vi "Save into new sequence.vi"(5 "To":u32, 7 "From":u32, 9 "Header2 file data":T1, 10 "Header file data":T2 {"Pixel depth" items=["8 bits", "16 bits", "Float", "Complex", "RGB", "HSL"]; "time of 1st frame, \nsec since 1/1/04" format="%.2f"}, 11 "Acquisition refnum array":refnum<file>[](array[refnum])) -> ()   [LabVIEW 2015]
uses:
  GLIMPSE Globals.vi
  Seq file v 1/Offset.ctl
  Seq file v 1/file number.ctl
  Seq file v 1/Offset table.ctl
  Header file data.ctl
  Header2 file data.ctl
panel:
  out "Output frame number 2":i32(slide) scale=0.0..68.0
  out "Input Sequences Progress (%) 2":dbl[](array[slide]) scale=0.0..100.0
  in  "error in":errorcluster
  out "Input Sequences Progress (%)":dbl[](array[slide]) scale=0.0..100.0
  out "Output frame number":i32(slide) scale=0.0..68.0
  out "Save into new directory:":path=path "d:/1.glimpse"
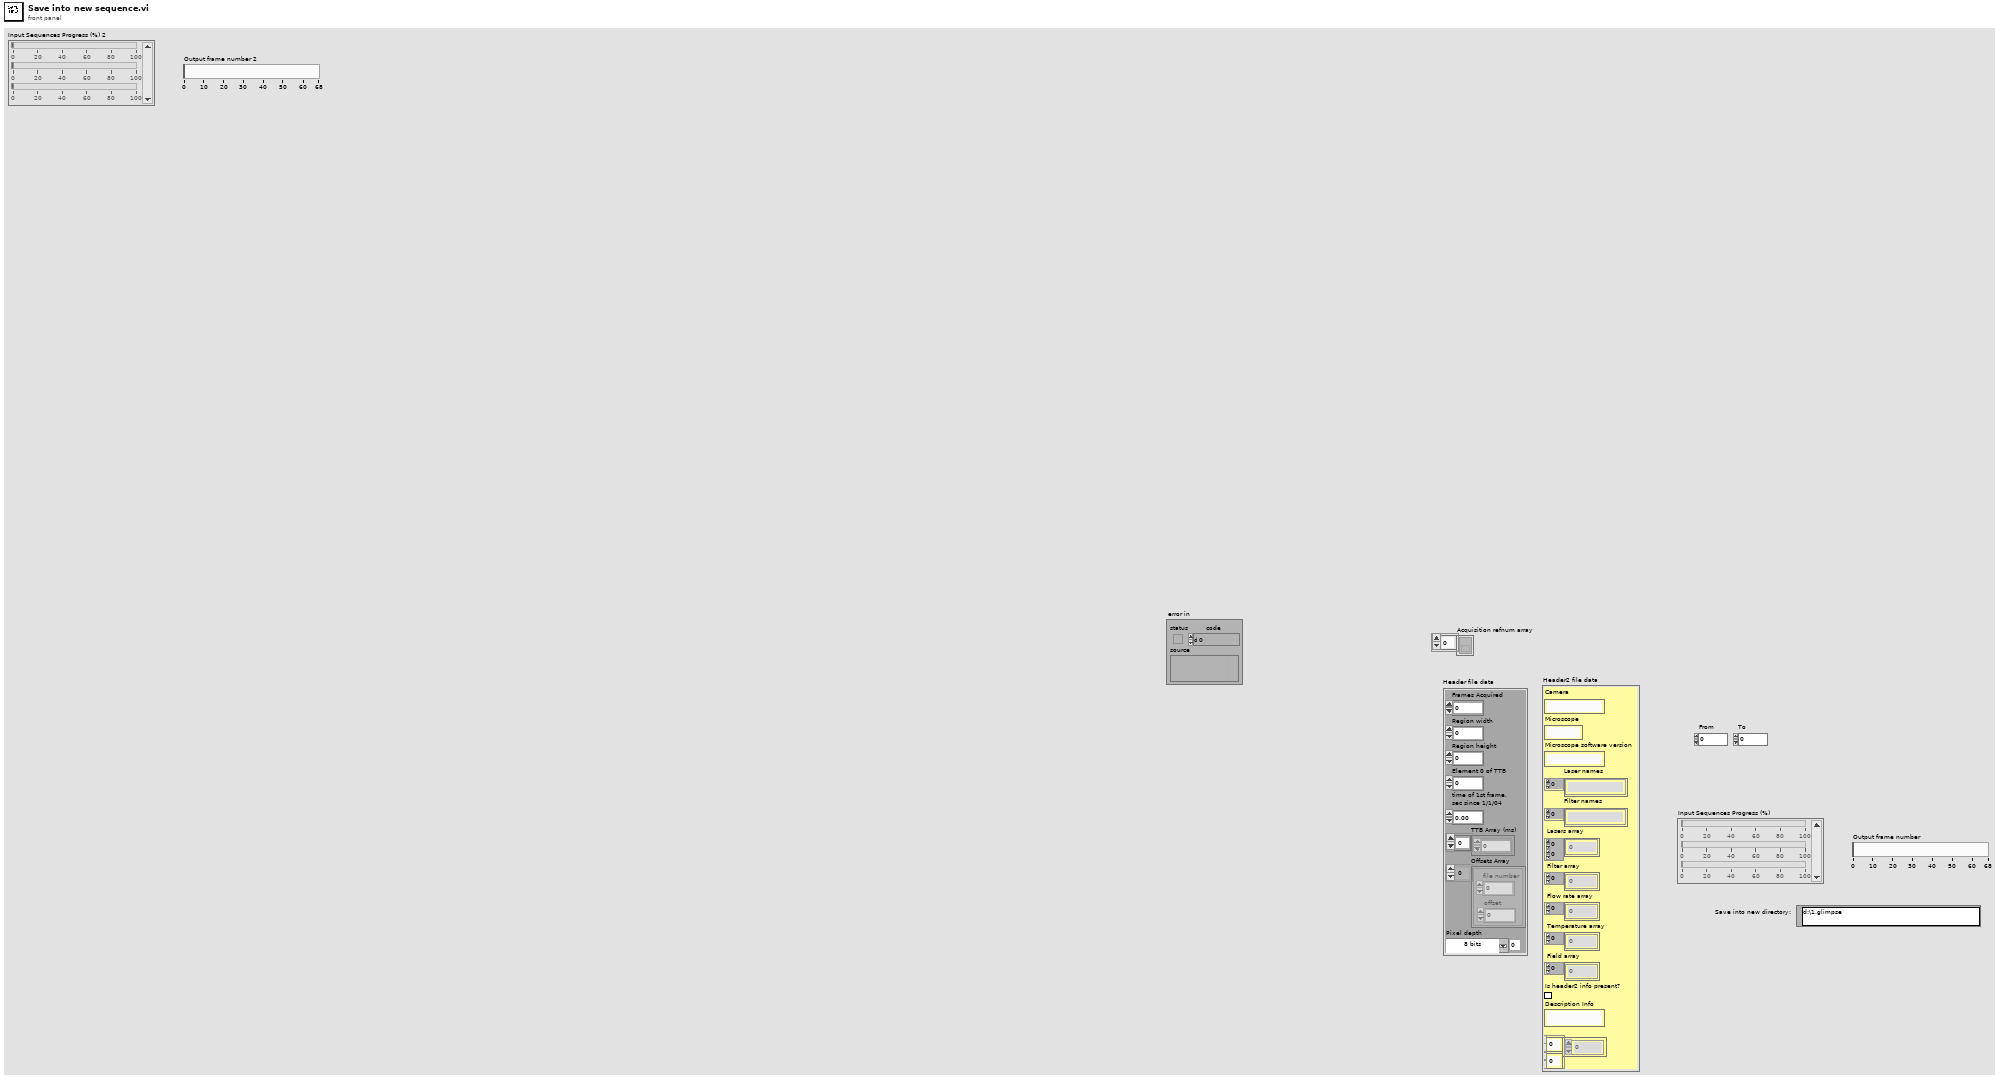
[diagram p1: front panel]
types:
  T1 = typedef "Header2 file data.ctl" = cluster{"Camera":string, "Microscope":string, "Microscope software version":string, "Laser names":string[], "Filter names":string[], "Lasers array":u16[][], "Filter array":u16[], "Flow rate array":dbl[], "Temperature array":dbl[], "Field array":u16[], "Is header2 info present?":bool, "Description Info":string, "Stage xyz array":dbl[][]}
  T2 = typedef "Header file data.ctl" = cluster{"Frames Acquired":u32, "Region width":i32, "Region height":i32, "Element 0 of TTB":u32, "time of 1st frame, \nsec since 1/1/04":dbl, "TTB Array (ms)":u32[], "Offsets Array":T3, "Pixel depth":u32}
  T3 = typedef "Offset table.ctl" = cluster{"offset":T4, "file number":T5}[]
  T4 = typedef "Offset.ctl" = i32
  T5 = typedef "file number.ctl" = u8
  T6 = typedef "Sequence files handle.ctt" = cluster{"Sequence files directory path":path, "Sequence files refnum array":refnum<file>[]}
  T7 = typedef "IMAQ Image.ctl" = refnum<image>
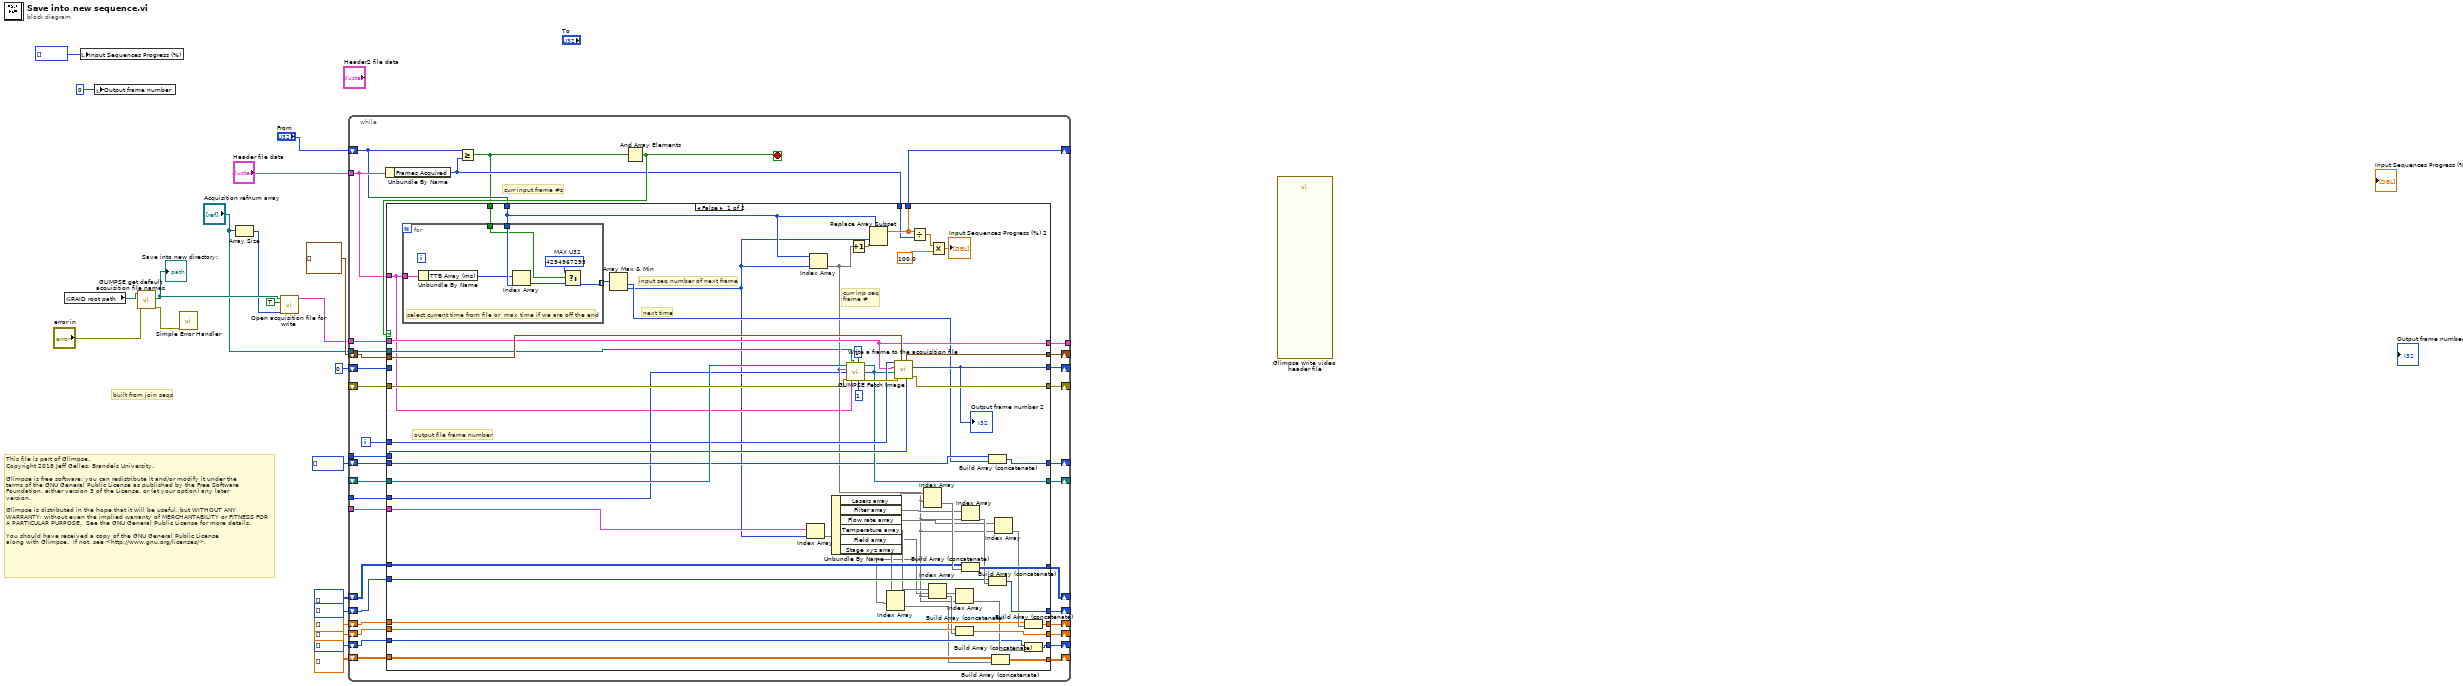
[diagram p0: block diagram]
diagram:
  # "built from join seqs"
  # "This file is part of Glimpse. \nCopyright 2018 Jeff Gelles, Brandeis University.    \n\nGlimpse is free software: you can redistribute it and/or modify it under the \nterms of the GNU General Public License as published by the Free Software \nFoundation, either version 3 of the License, or (at your option) any later \nversion.\n\nGlimpse is distributed in the hope that it will be useful, but WITHOUT ANY \nWARRANTY; without even the implied warranty of MERCHANTABILITY or FITNESS FOR \nA PARTICULAR PURPOSE.  See the GNU General Public License for more details.\n\nYou should have received a copy of the GNU General Public License\nalong with Glimpse.  If not, see <http://www.gnu.org/licenses/>."
  n1 = global read "GLIMPSE Globals.vi" "RAID root path"() -> (w25:path)
  n2 = local write "Input Sequences Progress (%)"(u64[] [] ("Input Sequences Progress (%)")) -> ()
  n3 = local write "Output frame number"(0 ("Output frame number")) -> ()
  n4 = call "GLIMPSE get default acquisition file names.vi"("error in"="error in", "RAID root path"=w25) -> ("error out"=w28:errorcluster, "next directory path"=w23:path)  [unwired: 6 out]
  "Save into new directory:" <- w23
  n5 = call <vilib>:"Simple Error Handler.vi"("error in (no error)"=w28) -> ()  [unwired: 1 in, 8 out]
  n6 = Array Size(array="Acquisition refnum array") -> (size(s)=w21:i32)
  n7 = call "Open acquisition file for write.vi"("Number of acquisition files"=w21, "Use new?"=TRUE, "New directory to create"=w23) -> ("Sequence files handle"=w2:T6)  [unwired: 1 in, 6 out]
  n8 = while {
    tunnel: "Header file data" -> [w62]
    shift-right: [w50] -> _
    shift-left: "From" -> [w61]
    tunnel: "Acquisition refnum array" -> [w60]
    shift-right: [w58] -> w14
    shift-left: _ -> [w59]
    shift-right: [w49] -> _
    shift-left: [w57] -> w20
    tunnel: w2 -> [w56]
    tunnel: [w54] -> w19
    shift-right: [w53] -> _
    shift-left: cluster{"offset":i32, "file number":u8}[] [] ("Offset table out") -> [w52]
    tunnel: [w51] -> w17
    shift-right: [w48] -> w13
    shift-left: u32[] [] -> [w47]
    shift-right: [w46] -> w12
    shift-left: u32 0 ("Last frame number written out") -> [w45]
    tunnel: [w44] -> _
    tunnel: [w42] -> w11
    shift-right: [w41] -> _
    shift-left: u16[][] [] -> [w40]
    shift-right: [w39] -> _
    shift-left: u16[] [] -> [w38]
    shift-right: [w37] -> _
    shift-left: dbl[] [] -> [w36]
    shift-right: [w35] -> _
    shift-left: dbl[] [] -> [w34]
    shift-right: [w33] -> _
    shift-left: u16[] [] -> [w32]
    shift-right: [w30] -> _
    shift-left: dbl[][] [] -> [w31]
    i -> [w55]
    stop <- w63 stop-if-true
    # "curr input frame #s"
    n9 = Unbundle By Name(w62) -> ("Frames Acquired"=w43:u32)
    n10 = Greater Or Equal?(x=w61, y=w43) -> (x >= y?=w29:bool)
    n11 = And Array Elements(Boolean array=w29) -> (logical AND=w63:bool)
    n12 = case shown="False" w63 {
      tunnel: w62 -> [w65 _]
      tunnel: w61 -> [w108 w133]
      tunnel: w60 -> [w66 _]
      tunnel: w59 -> [w118 w137]
      tunnel: [w113 w137] -> w58
      tunnel: w57 -> [w115 w135]
      tunnel: w56 -> [w103 w134]
      tunnel: w55 -> [w112 _]
      tunnel: w54 -> [w68 _]
      tunnel: [w111 w139] -> w53
      tunnel: w52 -> [w110 w139]
      tunnel: w51 -> [w109 _]
      tunnel: [w102 w133] -> w50
      tunnel: [w106 w135] -> w49
      tunnel: [w105 w136] -> w48
      tunnel: w47 -> [w104 w136]
      tunnel: [w97 w138] -> w46
      tunnel: w45 -> [_ w138]
      tunnel: [w103 w134] -> w44
      tunnel: w43 -> [w101 _]
      tunnel: w42 -> [w94 _]
      tunnel: [w91 w132] -> w41
      tunnel: w40 -> [w90 w132]
      tunnel: [w87 w131] -> w39
      tunnel: w38 -> [w86 w131]
      tunnel: [w77 w130] -> w37
      tunnel: w36 -> [w83 w130]
      tunnel: [w81 w129] -> w35
      tunnel: w34 -> [w79 w129]
      tunnel: [w76 w128] -> w33
      tunnel: w32 -> [w74 w128]
      tunnel: w31 -> [w73 w127]
      tunnel: [w69 w127] -> w30
      tunnel: w29 -> [w67 _]
      frame False {
        # "output file frame number"
        # "curr inp seq\nframe #"
        # "input seq number of next frame"
        # "next time"
        n13 = for {
          tunnel: w65 -> [w126]
          tunnel: w108 -> [w125]
          tunnel: [w122] -> w119 mode=indexing
          tunnel: w67 -> [w121]
          w120 = u32 4294967295  # MAX U32
          # "select current time from file or  max time if we are off the end"
          n14 = Unbundle By Name(w126) -> ("TTB Array (ms)"=w124:u32[])
          n15 = Index Array(array=w124, index=w125) -> (element=w123:u32)
          n16 = Select(t=w120, s=w121, f=w123) -> (s? t:f=w122:u32)
        }
        n17 = Array Max & Min(array=w119) -> (min value=w96:u32, min index (indices)=w64:i32)  [unwired: 2 out]
        n18 = Index Array(array=w94, index=w64) -> (element=w95)
        n19 = Index Array(array=w108, index=w64) -> (element=w71)
        n20 = Unbundle By Name(w95) -> ("Lasers array"=w93, "Filter array"=w89, "Flow rate array"=w85, "Temperature array"=w82, "Field array"=w78, "Stage xyz array"=w72)
        n21 = call "GLIMPSE Fetch Image.vi"("Display FOV number"=i16 1, "Total FOVs"=i16 1, "Header file data"=w65, "Acqisition files refnums"=w66, "error in"=w118, "Logical Frame Number\n(starting with zero)"=w71, "Image In"=w115) -> ("error out"=w114:errorcluster, "Image Out"=w106:T7)  [unwired: 2 in, 1 out]
        n22 = Increment(x=w71) -> (x+1=w107:dbl)
        n23 = Replace Array Subset(array=w108, new element=w107, index=w64) -> (w102:dbl[])
        n24 = Index Array(array=w72, index (row)=w71) -> (element=w70)  [unwired: 1 in]
        n25 = call "Write a frame to the acquisition file.vi"("Pixel depth"=w68, "Frames per acquisition file"=w109, "Offset table in"=w110, "error in"=w114, "Image In"=w106, "Sequence files handle"=w103, "Last frame number written in"=w112) -> ("error out"=w113:errorcluster, "Last frame number written out"=w97:u32, "Offset table out"=w111:T3)  [unwired: 2 out]
        "Output frame number 2" <- w97
        n26 = Divide(x=w102, y=w101) -> (x/y=w100:dbl[])
        n27 = Index Array(array=w93, index (row)=w71) -> (element=w92)  [unwired: 1 in]
        n28 = Index Array(array=w82, index=w71) -> (element=w80)
        n29 = Multiply(x=w100, y=100.0) -> (x*y=→"Input Sequences Progress (%) 2":dbl[])
        n30 = Index Array(array=w78, index=w71) -> (element=w75)
        n31 = Build Array (concatenate)(w79, w80) -> (w81:dbl[])
        n32 = Index Array(array=w89, index=w71) -> (element=w88)
        n33 = Build Array (concatenate)(w90, w92) -> (w91:u16[][])
        n34 = Build Array (concatenate)(w104, w96) -> (w105:u32[])
        n35 = Build Array (concatenate)(w86, w88) -> (w87:u16[])
        n36 = Build Array (concatenate)(w73, w70) -> (w69:dbl[][])
        n37 = Index Array(array=w85, index=w71) -> (element=w84)
        n38 = Build Array (concatenate)(w83, w84) -> (w77:dbl[])
        n39 = Build Array (concatenate)(w74, w75) -> (w76:u16[])
      }
      frame True {
      }
    }
  }
  n40 = call "Glimpse write video header file.vi"() -> ()  [unwired: 19 in, 1 out]
